vi "Rotate Polygon.vi"(10 "Angle":dbl, 11 "Input Polygon":cluster{dbl, dbl}[](array[cluster])) -> (3 "Output Polygon":cluster{dbl, dbl}[](array[cluster]))   [LabVIEW 2020]
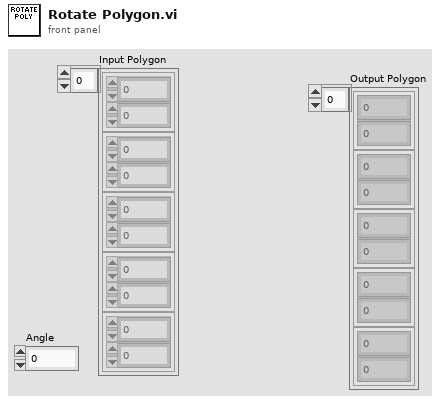
[diagram p1: front panel]
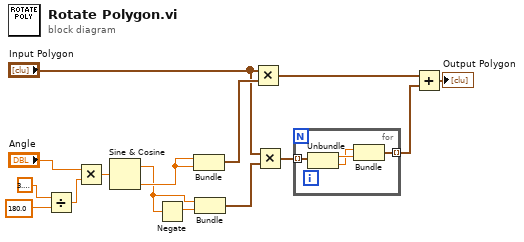
[diagram p0: block diagram]
diagram:
  n1 = Divide(x=3.141592653589793, y=180.0) -> (x/y=w12:dbl)
  n2 = Multiply(x="Angle", y=w12) -> (x*y=w10:dbl)
  n3 = Sine & Cosine(0:w10) -> (1:w4:dbl, 2:w6:dbl)
  n4 = Negate(x=w4) -> (-x=w5:dbl)
  n5 = Bundle(w6, w6) -> (w15:cluster{dbl, dbl})  [unwired: 1 in]
  n6 = Bundle(w4, w5) -> (w9:cluster{dbl, dbl})  [unwired: 1 in]
  n7 = Multiply(x="Input Polygon", y=w15) -> (x*y=w8:cluster{dbl, dbl}[])
  n8 = Multiply(x="Input Polygon", y=w9) -> (x*y=w3:cluster{dbl, dbl}[])
  n9 = for {
    tunnel: w3 -> [w19] mode=indexing
    tunnel: [w16] -> w2 mode=indexing
    n10 = Unbundle(w19) -> (w18:dbl, w17:dbl)
    n11 = Bundle(w17, w18) -> (w16:cluster{dbl, dbl})  [unwired: 1 in]
  }
  n12 = Add(x=w8, y=w2) -> (x+y=→"Output Polygon":cluster{dbl, dbl}[])
